vi "MecaDriveKinematicsConstraint_New.vi"(9 "MecanumKinematics":T1={"FrontLeft"={"X"=0.0, "Y"=0.0}, "FrontRight"={"X"=0.0, "Y"=0.0}, "RearLeft"={"X"=0.0, "Y"=0.0}, "RearRight"={"X"=0.0, "Y"=0.0}, "InverseKinematics"=[[0.0, 1.0, -1.0, 0.0], [0.0, 1.0, 1.0, 0.0], [0.0, 1.0, 1.0, 0.0], [0.0, 1.0, -1.0, 0.0]], "ForwardKinematics"=[[0.0, 1.0, -1.0, 0.0], [0.0, 1.0, 1.0, 0.0], [0.0, 1.0, 1.0, 0.0], [0.0, 1.0, -1.0, 0.0]], "PrevCoR"={"X"=0.0, "Y"=0.0}} {"PrevCoR"."Y" format="%14.3f"; "PrevCoR"."X" format="%14.3f"; "RearRight"."Y" format="%14.3f"; "RearRight"."X" format="%14.3f"; "RearLeft"."Y" format="%14.3f"; "RearLeft"."X" format="%14.3f"; "FrontRight"."Y" format="%14.3f"; "FrontRight"."X" format="%14.3f"; "FrontLeft"."Y" format="%14.3f"; "FrontLeft"."X" format="%14.3f"}, 11 "Max Speed (M/S)":dbl format="%20.4f") -> (3 "MECANUM_DRIVE_KINE_CONSTRAINT":T4={"Max Speed (M/S)"=0.0, "MECA_DRIVE_KINEMATICS"={"FrontLeft"={"X"=0.0, "Y"=0.0}, "FrontRight"={"X"=0.0, "Y"=0.0}, "RearLeft"={"X"=0.0, "Y"=0.0}, "RearRight"={"X"=0.0, "Y"=0.0}, "InverseKinematics"=[[0.0, 1.0, -1.0, 0.0], [0.0, 1.0, 1.0, 0.0], [0.0, 1.0, 1.0, 0.0], [0.0, 1.0, -1.0, 0.0]], "ForwardKinematics"=[[0.0, 1.0, -1.0, 0.0], [0.0, 1.0, 1.0, 0.0], [0.0, 1.0, 1.0, 0.0], [0.0, 1.0, -1.0, 0.0]], "PrevCoR"={"X"=0.0, "Y"=0.0}}} {"MECA_DRIVE_KINEMATICS"."PrevCoR"."Y" format="%14.3f"; "MECA_DRIVE_KINEMATICS"."PrevCoR"."X" format="%14.3f"; "MECA_DRIVE_KINEMATICS"."RearRight"."Y" format="%14.3f"; "MECA_DRIVE_KINEMATICS"."RearRight"."X" format="%14.3f"; "MECA_DRIVE_KINEMATICS"."RearLeft"."Y" format="%14.3f"; "MECA_DRIVE_KINEMATICS"."RearLeft"."X" format="%14.3f"; "MECA_DRIVE_KINEMATICS"."FrontRight"."Y" format="%14.3f"; "MECA_DRIVE_KINEMATICS"."FrontRight"."X" format="%14.3f"; "MECA_DRIVE_KINEMATICS"."FrontLeft"."Y" format="%14.3f"; "MECA_DRIVE_KINEMATICS"."FrontLeft"."X" format="%14.3f"; "Max Speed (M/S)" format="%20.4f"})   [LabVIEW 2019, in "Trajectory_Library.lvlib"]
doc: "Constructs a mecanum drive dynamics constraint.\n\nParameters:\n - maxVelocity - Maximum allowed velocity.\n - MecanumDriveKinematics - Data structure\n\nReturns\n - MecanumDriveKinematicsConstraint - Constraint data structure"
uses:
  Trajectory_Library.lvlib
  TRAJ_CONSTRAINT_MECA_DRIVE_KINEMATICS.ctl
  MECA_DRIVE_KINEMATICS.ctl
  TRANSLATION2D.ctl
  <vilib>/Analysis/Matrix/Datatypes/RealMatrix.ctl
  <vilib>/Analysis/Matrix/NI_Matrix.lvlib
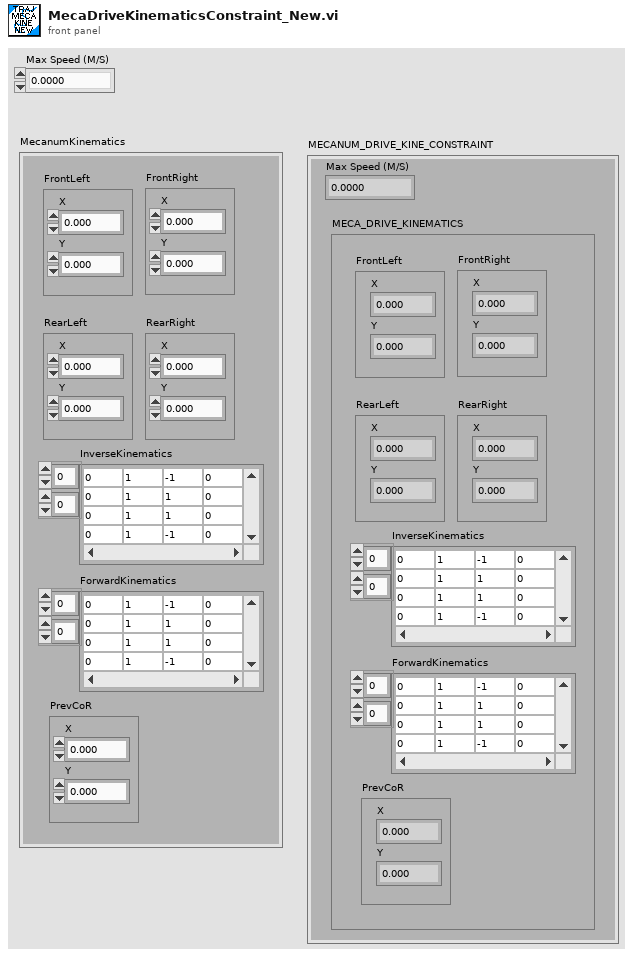
[diagram p1: front panel]
types:
  T1 = typedef "Trajectory_Library.lvlib/MECA_DRIVE_KINEMATICS.ctl" = cluster{"FrontLeft":T2, "FrontRight":T2, "RearLeft":T2, "RearRight":T2, "InverseKinematics":T3, "ForwardKinematics":T3, "PrevCoR":T2}
  T2 = typedef "Trajectory_Library.lvlib/TRANSLATION2D.ctl" = cluster{"X":dbl, "Y":dbl}
  T3 = typedef "NI_Matrix.lvlib/RealMatrix.ctl" = dbl[][]
  T4 = typedef "Trajectory_Library.lvlib/TRAJ_CONSTRAINT_MECA_DRIVE_KINEMATICS.ctl" = cluster{"Max Speed (M/S)":dbl, "MECA_DRIVE_KINEMATICS":T1}
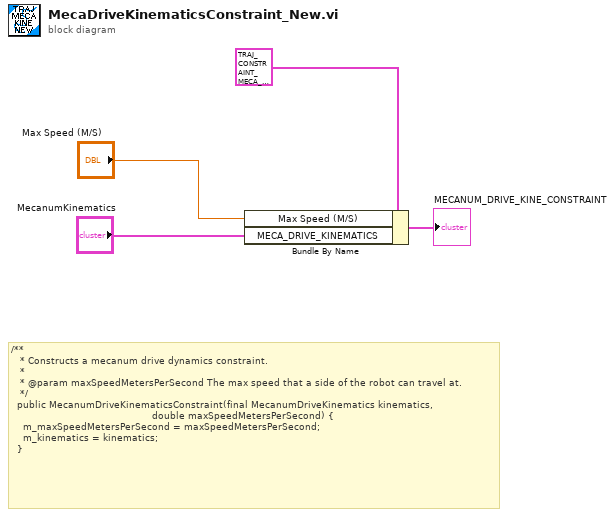
[diagram p0: block diagram]
diagram:
  # "/**\n   * Constructs a mecanum drive dynamics constraint.\n   *\n   * @param maxSpeedMetersPerSecond The max speed that a side of the robot can travel at.\n   */\n  public MecanumDriveKinematicsConstraint(final MecanumDriveKinematics kinematics,\n                                               double maxSpeedMetersPerSecond) {\n    m_maxSpeedMetersPerSecond = maxSpeedMetersPerSecond;\n    m_kinematics = kinematics;\n  }"
  n1 = Bundle By Name(cluster=T4 {"Max Speed (M/S)"=0.0, "MECA_DRIVE_KINEMATICS"={"FrontLeft"={"X"=0.0, "Y"=0.0}, "FrontRight"={"X"=0.0, "Y"=0.0}, "RearLeft"={"X"=0.0, "Y"=0.0}, "RearRight"={"X"=0.0, "Y"=0.0}, "InverseKinematics"=[[0.0, 1.0, -1.0, 0.0], [0.0, 1.0, 1.0, 0.0], [0.0, 1.0, 1.0, 0.0], [0.0, 1.0, -1.0, 0.0]], "ForwardKinematics"=[[0.0, 1.0, -1.0, 0.0], [0.0, 1.0, 1.0, 0.0], [0.0, 1.0, 1.0, 0.0], [0.0, 1.0, -1.0, 0.0]], "PrevCoR"={"X"=0.0, "Y"=0.0}}} ("MECANUM_DRIVE_KINE_CONSTRAINT"), "Max Speed (M/S)"="Max Speed (M/S)", "MECA_DRIVE_KINEMATICS"="MecanumKinematics") -> (→"MECANUM_DRIVE_KINE_CONSTRAINT":T4)
